vi "Battery model function and gradient.vi"(3 "output control":T1, 4 "data":variant, 5 "X":dbl[](array[numeric]), 6 "a":dbl[](array[numeric])) -> (0 "error out":errorcluster, 1 "f'(X,a)":dbl[][](array[numeric]), 2 "f(X,a)":dbl[](array[numeric]))   [LabVIEW 2013]
doc: "This template is the starting point for creating a model function to be passed to the Nonlinear Curve Fit.vi."
uses:
  <vilib>/gmath/NumericalOptimization/LM_output select.ctl
  <vilib>/imath/engines/lvmath2/RunTimeEngine/ErrorHandling/NIMS_Finalize Error.vi
  <vilib>/imath/engines/lvmath2/RunTimeEngine/IndexRead/NIMS V(S).vi
  <instcachedir>/0/NIMS V(S)_0488751826AF41519A22953C041130DC.lvgen/NIMS V(S)_0488751826AF41519A22953C041130DC_000.vi
  <vilib>/imathl/engines/lvmath/Functions/Error Handling/Create Error.vi
  <vilib>/imath/engines/lvmath2/RunTimeEngine/NodeEndStatement/NIMS_NodeEndStatement_Output.vi
  <instcachedir>/0/NIMS_NodeEndStatement_Output_53EC0D466D134D7ABD903AC30B43404B.lvgen/NIMS_NodeEndStatement_Output_53EC0D466D134D7ABD903AC30B43404B_000.vi
  <instcachedir>/0/NIMS_NodeEndStatement_Output_53EC0D466D134D7ABD903AC30B43404B.lvgen/NIMS_NodeEndStatement_Output_53EC0D466D134D7ABD903AC30B43404B_009.vi
  <vilib>/imath/engines/lvmath2/RunTimeEngine/IndexReplace/NIMS V(S)=S.vi
  <instcachedir>/0/NIMS V(S)=S_66A18068148B4981A312229A93EA5C06.lvgen/NIMS V(S)=S_66A18068148B4981A312229A93EA5C06_001.vi
  <vilib>/imath/engines/lvmath2/RunTimeEngine/ArithmeticOperatorToken/NIMS_ArithmeticOperator_power(S).vi
  <instcachedir>/0/NIMS_ArithmeticOperator_power(S)_7602F12E697C47D8910FAD43BB85D848.lvgen/NIMS_ArithmeticOperator_power(S)_7602F12E697C47D8910FAD43BB85D848_010.vi
  <vilib>/imath/engines/lvmath2/RunTimeEngine/ErrorHandling/NIMS_Create Error From Enums.vi
  <vilib>/gmath/NI_Gmath.lvlib
panel:
  out "XY Graph":cluster{dbl[], dbl[]}(graph)
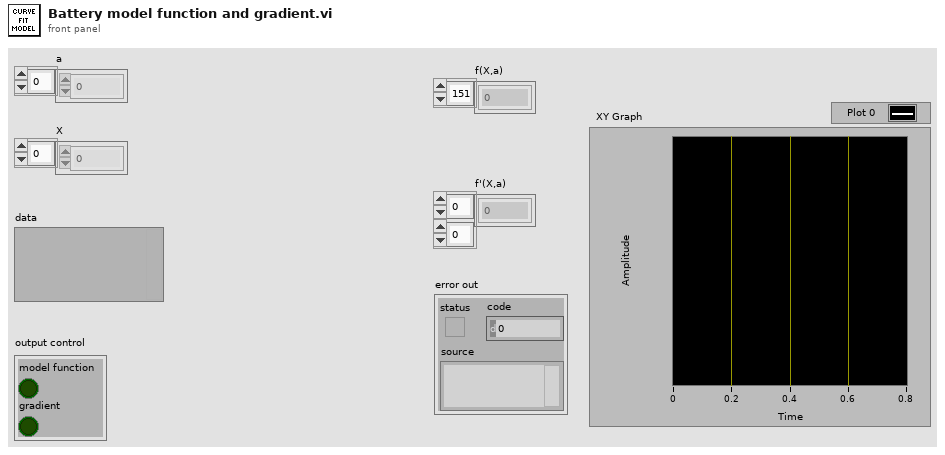
[diagram p1: front panel]
types:
  T1 = typedef "NI_Gmath.lvlib/LM_output select.ctl" = cluster{"model function":bool, "gradient":bool}
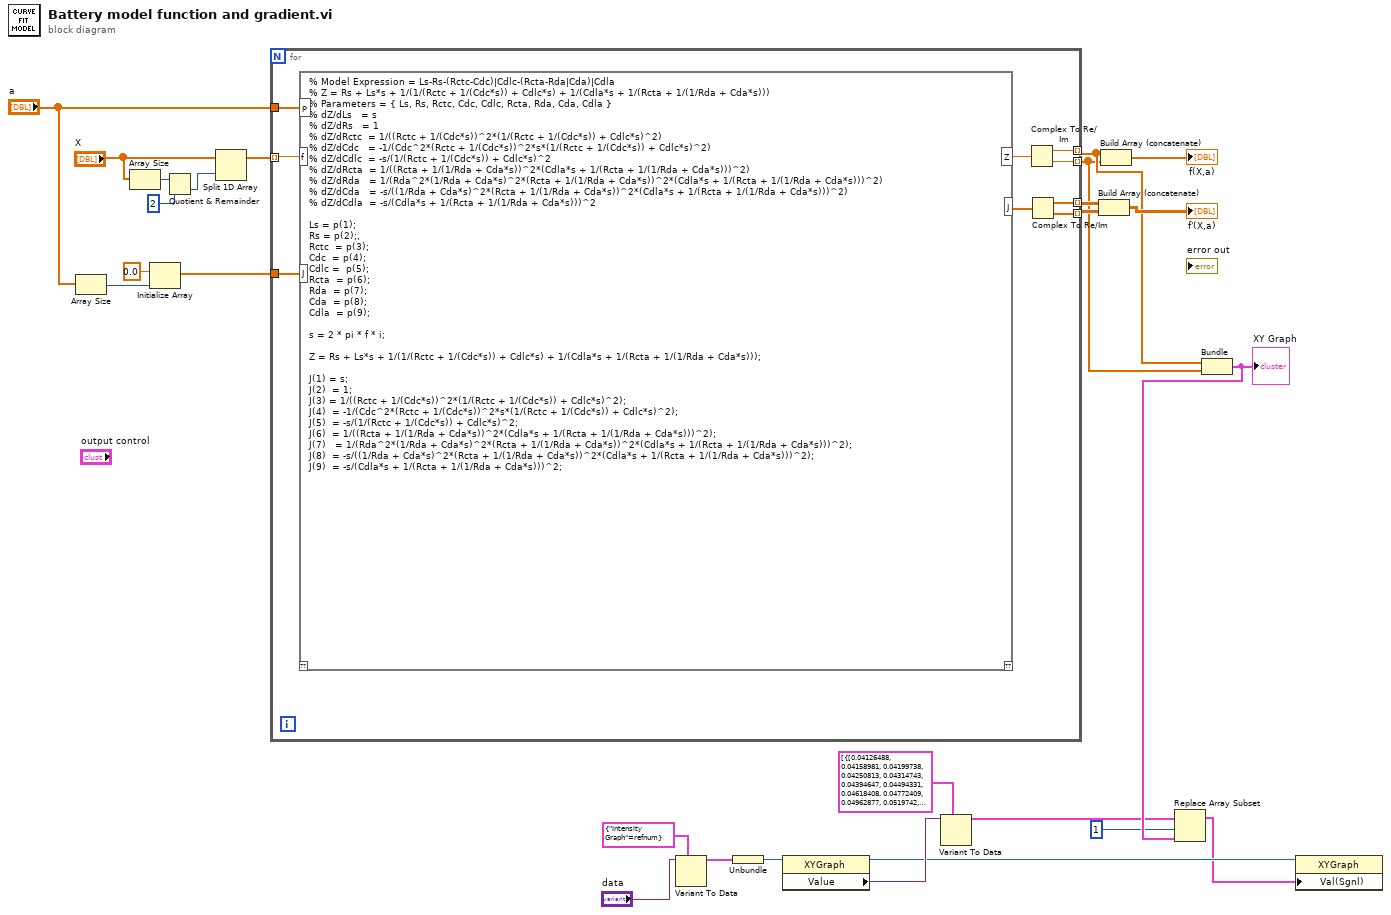
[diagram p0: block diagram]
diagram:
  n1 = Array Size(array="a") -> (size(s)=w20:i32)
  n2 = Array Size(array="X") -> (size(s)=w24:i32)
  n3 = Initialize Array(0.0 ("element"), w20) -> (w18:dbl[])
  n4 = Quotient & Remainder(x=w24, y=2) -> (floor(x/y)=w22:i32)  [unwired: 1 out]
  n5 = Split 1D Array(array="X", index=w22) -> (first subarray=w26:dbl[])  [unwired: 1 out]
  n6 = for {
    tunnel: "a" -> [w35]
    tunnel: w26 -> [w34] mode=indexing
    tunnel: w18 -> [w33]
    tunnel: [w30] -> w13 mode=indexing
    tunnel: [w29] -> w12 mode=indexing
    tunnel: [w28] -> w16 mode=indexing
    tunnel: [w27] -> w15 mode=indexing
    n7 = mathscript code="% Model Expression = Ls-Rs-(Rctc-Cdc)|Cdlc-(Rcta-Rda|Cda)|Cdla\n% Z = Rs + Ls*s + 1/(1/(Rctc + 1/(Cdc*s)) + Cdlc*s) + 1/(Cdla*s + 1/(Rcta + 1/(1/Rda + Cda*s)))\n% Parameters = { Ls, Rs, Rctc, Cdc, Cdlc, Rcta, Rda, Cda, Cdla }\n% dZ/dLs \t = s\n% dZ/dRs \t = 1\n% dZ/dRctc  = 1/((Rctc + 1/(Cdc*s))^2*(1/(Rctc + 1/(Cdc*s)) + Cdlc*s)^2)\n% dZ/dCdc \t = -1/(Cdc^2*(Rctc + 1/(Cdc*s))^2*s*(1/(Rctc + 1/(Cdc*s)) + Cdlc*s)^2)\n% dZ/dCdlc  = -s/(1/(Rctc + 1/(Cdc*s)) + Cdlc*s)^2\n% dZ/dRcta  = 1/((Rcta + 1/(1/Rda + Cda*s))^2*(Cdla*s + 1/(Rcta + 1/(1/Rda + Cda*s)))^2)\n% dZ/dRda \t = 1/(Rda^2*(1/Rda + Cda*s)^2*(Rcta + 1/(1/Rda + Cda*s))^2*(Cdla*s + 1/(Rcta + 1/(1/Rda + Cda*s)))^2)\n% dZ/dCda \t = -s/((1/Rda + Cda*s)^2*(Rcta + 1/(1/Rda + Cda*s))^2*(Cdla*s + 1/(Rcta + 1/(1/Rda + Cda*s)))^2)\n% dZ/dCdla  = -s/(Cdla*s + 1/(Rcta + 1/(1/Rda + Cda*s)))^2\n\nLs = p(1);\nRs = p(2);, \nRctc  = p(3);\nCdc  = p(4);\nCdlc =  p(5);\nRcta  = p(6);\nRda  = p(7);\nCda  = p(8);\nCdla  = p(9);\n\ns = 2 * pi * f * i;\n\nZ = Rs + Ls*s + 1/(1/(Rctc + 1/(Cdc*s)) + Cdlc*s) + 1/(Cdla*s + 1/(Rcta + 1/(1/Rda + Cda*s)));\n\nJ(1) = s;\nJ(2)\t = 1;\nJ(3) = 1/((Rctc + 1/(Cdc*s))^2*(1/(Rctc + 1/(Cdc*s)) + Cdlc*s)^2);\nJ(4)\t = -1/(Cdc^2*(Rctc + 1/(Cdc*s))^2*s*(1/(Rctc + 1/(Cdc*s)) + Cdlc*s)^2);\nJ(5)  = -s/(1/(Rctc + 1/(Cdc*s)) + Cdlc*s)^2;\nJ(6)  = 1/((Rcta + 1/(1/Rda + Cda*s))^2*(Cdla*s + 1/(Rcta + 1/(1/Rda + Cda*s)))^2);\nJ(7) \t = 1/(Rda^2*(1/Rda + Cda*s)^2*(Rcta + 1/(1/Rda + Cda*s))^2*(Cdla*s + 1/(Rcta + 1/(1/Rda + Cda*s)))^2);\nJ(8)\t = -s/((1/Rda + Cda*s)^2*(Rcta + 1/(1/Rda + Cda*s))^2*(Cdla*s + 1/(Rcta + 1/(1/Rda + Cda*s)))^2);\nJ(9)  = -s/(Cdla*s + 1/(Rcta + 1/(1/Rda + Cda*s)))^2;"("p"=w35, "f"=w34, "J"=w33) -> ("Z"=w31:cdb, "J"=w32:cdb[])  [unwired: 1 in, 1 out]
    n8 = Complex To Re/Im(x + iy=w31) -> (x=w30:dbl, y=w29:dbl)
    n9 = Complex To Re/Im(x + iy=w32) -> (x=w28:dbl[], y=w27:dbl[])
  }
  n10 = Variant To Data(type=cluster{"Intensity Graph":refnum<vi>} {"Intensity Graph"=refnum} ("output cluster"), Variant="data") -> (data=w10:cluster{"Intensity Graph":refnum<vi>})  [unwired: 1 in, 1 out]
  n11 = Unbundle(w10) -> ("Intensity Graph"=w6:refnum<vi>)
  n12 = property class="XYGraph"(reference=w6) -> (reference out=w2:refnum<vi>, "Value"=w5:variant)  [unwired: 1 in, 1 out]
  n13 = Variant To Data(type=cluster{dbl[], dbl[]}[] [{[0.04126488, 0.04158981, 0.04199738, 0.04250813, 0.04314743, 0.04394647, 0.04494331, 0.04618408, 0.04772409, 0.04962877, 0.0519742, 0.0548469, 0.05834239, 0.06256184, 0.06760643, 0.07356869, 0.08052083, 0.08850068, 0.09749691, 0.1074364, 0.1181775, 0.1295128, 0.141183, 0.1529012, 0.1643841, 0.175382, 0.1857037, 0.1952307, 0.2039205, 0.2118007, 0.218958, 0.2255252, 0.2316687, 0.2375799, 0.2434684, 0.2495579, 0.2560848, 0.2632954, 0.2714434, 0.2807835, 0.291561, 0.3039956, 0.3182595, 0.3344495, 0.3525587, 0.3724514, 0.3938493, 0.416337, 0.4393888, 0.4624172, 0.4848327, 0.5061048, 0.5258096, 0.5436572, 0.5594965, 0.5733007, 0.5851424, 0.5951632, 0.6035461, 0.6104913, 0.6161994, 0.6208601, 0.6246451, 0.6277055, 0.6301713, 0.6321524, 0.6337403, 0.6350109, 0.6360259, 0.636836, 0.6374817, 0.6379962, 0.6384058, 0.6387317, 0.638991, 0.6391972, 0.6393612, 0.6394915, 0.6395951, 0.6396774, 0.6397428, 0.6397948, 0.6398361, 0.639869, 0.639895, 0.6399158, 0.6399323, 0.6399454, 0.6399558, 0.6399642, 0.6399708, 0.6399761, 0.6399804, 0.6399839, 0.6399868, 0.6399892, 0.6399913, 0.6399931, 0.6399948, 0.6399964, 0.6399981, 0.64, 0.640002, 0.6400044, 0.6400073, 0.6400108, 0.6400151, 0.6400205, 0.6400272, 0.6400355, 0.640046, 0.6400592, 0.6400757, 0.6400965, 0.6401227, 0.6401557, 0.6401971, 0.6402493, 0.640315, 0.6403977, 0.6405017, 0.6406325, 0.6407972, 0.6410044, 0.6412649, 0.6415925, 0.6420043, 0.6425218, 0.6431718, 0.6439876, 0.6450108, 0.6462931, 0.6478979, 0.6499034, 0.6524051, 0.6555185, 0.6593819, 0.664159, 0.6700395, 0.6772392, 0.6859954], [0.2967524, 0.2604928, 0.2277047, 0.197959, 0.1708694, 0.1460881, 0.1233026, 0.1022327, 0.08262973, 0.06427518, 0.04698188, 0.03059545, 0.01499719, 0.0001075807, -0.01410996, -0.02764623, -0.04044574, -0.0524103, -0.06340858, -0.07329263, -0.08192073, -0.08918393, -0.09503155, -0.09948971, -0.1026685, -0.1047558, -0.1059995, -0.1066836, -0.1071023, -0.1075386, -0.1082484, -0.1094519, -0.1113294, -0.1140211, -0.1176284, -0.1222139, -0.1278009, -0.1343701, -0.1418538, -0.1501279, -0.1590041, -0.1682222, -0.1774476, -0.1862767, -0.1942534, -0.2009005, -0.2057633, -0.2084605, -0.2087338, -0.206484, -0.2017841, -0.1948662, -0.1860854, -0.1758711, -0.164675, -0.1529281, -0.1410095, -0.1292303, -0.1178289, -0.1069753, -0.09677938, -0.08730281, -0.07856953, -0.07057593, -0.06329917, -0.05670382, -0.05074691, -0.04538168, -0.04056024, -0.03623533, -0.03236156, -0.02889609, -0.02579904, -0.02303367, -0.02056638, -0.01836662, -0.01640677, -0.01466193, -0.01310973, -0.01173014, -0.01050524, -0.009419061, -0.008457384, -0.007607591, -0.006858504, -0.006200255, -0.005624158, -0.005122605, -0.004688965, -0.004317501, -0.004003298, -0.003742194, -0.003530732, -0.00336611, -0.003246146, -0.003169251, -0.003134406, -0.003141149, -0.003189571, -0.003280314, -0.003414583, -0.003594159, -0.003821424, -0.004099394, -0.004431755, -0.004822915, -0.005278063, -0.005803234, -0.00640539, -0.007092515, -0.007873714, -0.008759339, -0.009761117, -0.01089231, -0.01216788, -0.0136047, -0.01522173, -0.01704032, -0.01908441, -0.02138087, -0.02395982, -0.02685498, -0.03010405, -0.03374916, -0.03783725, -0.04242059, -0.0475572, -0.0533113, -0.05975371, -0.06696214, -0.07502134, -0.08402302, -0.09406533, -0.1052519, -0.1176902, -0.1314886, -0.1467524, -0.1635787, -0.1820481, -0.2022158, -0.2241001]}, {[0.04126487685962032, 0.04158980847691639, 0.0419973804922247, 0.04250813216274564, 0.04314743470540475, 0.0439464667760118, 0.04494330719873761, 0.046184080925646624, 0.047724090834876956, 0.04962876612476469, 0.051974192942764987, 0.0548469021932835, 0.0583423915848213, 0.06256183713554704, 0.06760643220936773, 0.07356869641114024, 0.08052083286013516, 0.08850065408217553, 0.09749693199100645, 0.10743643028098689, 0.11817751839658606, 0.12951281368868045, 0.14118296684961265, 0.1529012372451997, 0.1643841331746651, 0.1753820151951218, 0.1857036982725582, 0.19523067729682925, 0.20392044052209066, 0.21180067191657662, 0.21895801935412945, 0.22552514544559968, 0.23166869756550174, 0.2375799240591818, 0.24346835850505777, 0.24955792868610494, 0.25608478955713376, 0.26329539169360167, 0.2714434339397057, 0.2807835137423525, 0.2915609554008981, 0.30399563579284555, 0.31825950098747147, 0.3344495116438217, 0.3525587429673065, 0.3724513728612602, 0.3938493038097392, 0.4163369747665884, 0.4393888184466881, 0.4624171713865442, 0.4848326529019746, 0.506104748006444, 0.5258095936711688, 0.5436572306447477, 0.5594964846033067, 0.573300713834014, 0.5851423730561777, 0.5951632120990255, 0.6035461011173664, 0.6104912754616556, 0.6161994232490857, 0.6208601076656155, 0.6246450947302558, 0.6277055030530916, 0.6301713061567182, 0.6321523663323038, 0.6337403356414317, 0.6350108741049396, 0.6360259425948216, 0.6368359569911282, 0.6374817331900244, 0.6379961885867279, 0.6384057835315382, 0.6387317360017705, 0.6389910300611781, 0.639197235637379, 0.6393611833953078, 0.6394915091008094, 0.639595094357896, 0.6396774158250511, 0.6397428337922549, 0.6397948174134922, 0.639836125156094, 0.6398689507811932, 0.6398950386229368, 0.639915775484137, 0.6399322641975501, 0.6399453818701798, 0.6399558264804461, 0.6399641538631584, 0.6399708072252981, 0.6399761407468234, 0.639980438355287, 0.6399839288400901, 0.6399867980610396, 0.6399891987832753, 0.6399912588362802, 0.6399930879141642, 0.6399947834366072, 0.6399964356658008, 0.6399981325860862, 0.6399999645738861, 0.6400020291762051, 0.6400044363314249, 0.6400073142220162, 0.6400108160796965, 0.6400151283648121, 0.6400204806665974, 0.6400271579422334, 0.6400355156649536, 0.640045998702531, 0.6400591650345935, 0.640075715334612, 0.6400965301227581, 0.640122716726552, 0.6401556676983374, 0.6401971346546802, 0.6402493208601838, 0.6403149984821923, 0.6403976519996883, 0.6405016634453631, 0.6406325419610396, 0.6407972082962929, 0.6410043545303565, 0.6412648907182683, 0.6415924982265655, 0.6420043193744783, 0.6425218035179929, 0.6431717496819958, 0.6439875727756759, 0.645010829852108, 0.646293048013947, 0.6478978518016547, 0.649903400366849, 0.6524051149433328, 0.6555185023779543, 0.6593819347911429, 0.664158947650157, 0.6700395488256758, 0.6772392474538687, 0.6859953556245477], [0.2967524306083091, 0.26049280343467723, 0.2277046731337981, 0.19795898022839786, 0.17086936117979853, 0.1460881089082734, 0.12330255938485533, 0.10223275426465685, 0.08262975768782277, 0.06427520239664601, 0.046981903262358134, 0.030595460964158296, 0.014997173213383536, 0.00010758287565814772, -0.014109967454755712, -0.02764625188718148, -0.04044574742281566, -0.05241025779599622, -0.063408605193115, -0.0732926607840021, -0.08192072321292641, -0.08918393159132981, -0.09503154637648525, -0.09948970655086037, -0.10266850338232605, -0.1047557768129688, -0.10599953719388741, -0.10668362163887068, -0.1071023147509145, -0.10753857113074922, -0.10824841889226394, -0.10945190963135545, -0.11132939092535665, -0.11402114178320041, -0.11762838651038923, -0.12221387414806151, -0.1278009148122881, -0.13437011425327453, -0.14185377609516212, -0.15012791375608545, -0.15900407870001648, -0.16822220346504263, -0.17744765170786556, -0.1862766739806345, -0.19425338435952172, -0.20090053747789585, -0.205763299689201, -0.20846046238545632, -0.20873379305100703, -0.2064840192722472, -0.2017841194675794, -0.19486616114153119, -0.18608541604071505, -0.1758711029490645, -0.16467502089537078, -0.1529280471321538, -0.14100944216405867, -0.12923030606248015, -0.11782891605766709, -0.10697523007336962, -0.09677937786183838, -0.08730280335001749, -0.07856952594631658, -0.07057593532142946, -0.06329917161020217, -0.05670381711886597, -0.05074690299312099, -0.0453816816852312, -0.04056024129641725, -0.0362353347642086, -0.03236156759138129, -0.02889609336883478, -0.025799039324989132, -0.02303367052926025, -0.02056637398540664, -0.018366614773259213, -0.016406767196118218, -0.01466193442726198, -0.01310972972785703, -0.011730137261919635, -0.010505242248509322, -0.00941906093380097, -0.008457383991336416, -0.007607591041516942, -0.006858503778103756, -0.006200254575891037, -0.00562415771511992, -0.005122604787296614, -0.004688964837777946, -0.004317501272066441, -0.004003298226053895, -0.0037421945352909443, -0.0035307320627127447, -0.0033661098983032013, -0.0032461459136280714, -0.0031692507707461117, -0.0031344055995258776, -0.0031411487826836317, -0.0031895709071287663, -0.003280314395332614, -0.003414582879346358, -0.003594158864138815, -0.0038214241731744994, -0.004099393492953979, -0.004431754593935104, -0.004822914993372541, -0.0052780628773707065, -0.005803233136377128, -0.006405389361538614, -0.007092514325962369, -0.00787371311927286, -0.008759337794611242, -0.009761117561207774, -0.0108923096327048, -0.01216788417730132, -0.013604701620752427, -0.015221735557765355, -0.017040312942678104, -0.019084411260746614, -0.021380874074234783, -0.023959816055902715, -0.026854976362960886, -0.030104052242429485, -0.03374915561013425, -0.03783725244193273, -0.04242059274332402, -0.04755720268524233, -0.053311296942997626, -0.05975369938782436, -0.06696212957395983, -0.07502132846671639, -0.08402301072450001, -0.09406534239880271, -0.10525192681473082, -0.11769020212039227, -0.13148856472233827, -0.14675243162649848, -0.1635786236726158, -0.18204813643380693, -0.20221588522365946, -0.22410004353747742]}] ("XY Graph"), Variant=w5) -> (data=w3:cluster{dbl[], dbl[]}[])  [unwired: 1 in, 1 out]
  n14 = Build Array (concatenate)(w16, w15) -> (→"f'(X,a)":dbl[][])
  n15 = Build Array (concatenate)(w13, w12) -> (→"f(X,a)":dbl[])
  n16 = Bundle(w13, w12) -> (w11:cluster{dbl[], dbl[]})  [unwired: 1 in]
  "XY Graph" <- w11
  n17 = Replace Array Subset(array=w3, new element=w11, index=1) -> (w1:cluster{dbl[], dbl[]}[])
  n18 = property class="XYGraph"(reference=w2, "Val(Sgnl)"=w1) -> ()  [unwired: 1 in, 2 out]
